vi "set_switch.vi"(8 "error in (no error)":errorcluster {"code" format="%.0x"}, 9 "switch":i32, 10 "topology name":T1="1127/2-Wire 32x1 Mux", 11 "resource name":refnum<k15>="SR" caption="switcher resource name") -> (0 "error out":errorcluster)   [LabVIEW 2016]
uses:
  <instrlib>/niSwitch/niSwitch.LLB/niSwitch Topologies.ctl
  <vilib>/DAQmx/configure/hardwareSpecific/Switch.llb/DAQmx Switch Connect (Single).vi
panel:
  out "Pixel Set?":bool
  out "instrument handle out":refnum<k15>="SC1Mod2 (7)"
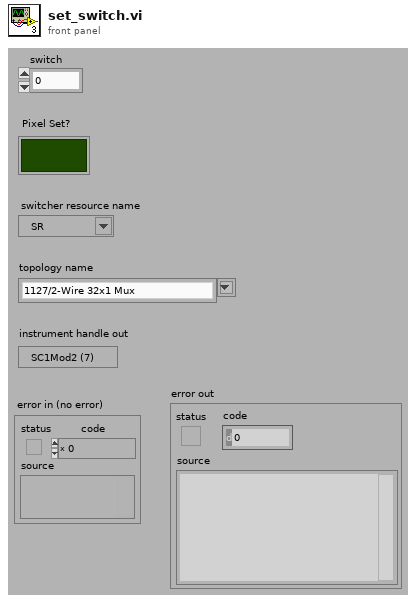
[diagram p1: front panel]
types:
  T1 = typedef "niSwitch Topologies.ctl" = string
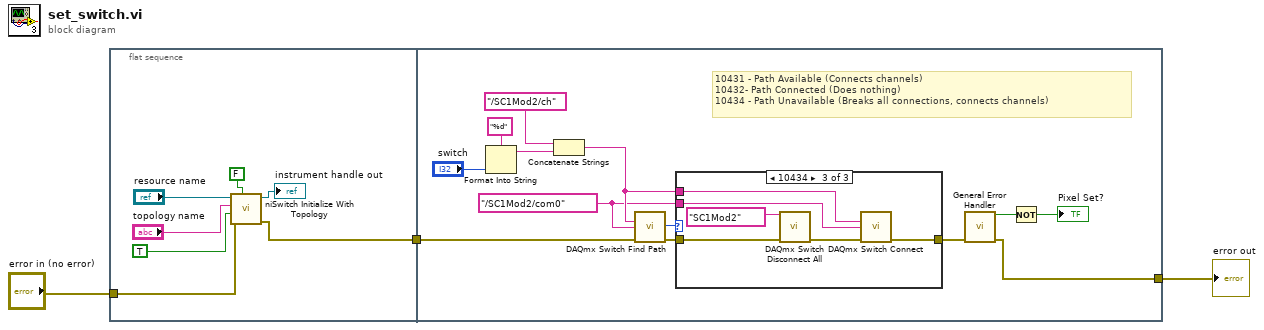
[diagram p0: block diagram]
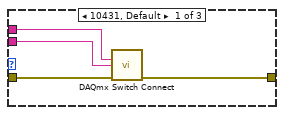
[diagram p2: hidden frame]
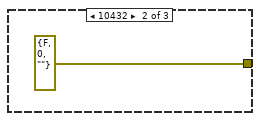
[diagram p3: hidden frame]
diagram:
  n1 = flat-sequence {
    tunnel: [w5] -> w3
    tunnel: "error in (no error)" -> [w4]
    tunnel: w3 -> [w12]
    tunnel: [w11] -> w1
    frame #0 {
      n2 = call <instrlib>:"niSwitch Initialize With Topology.vi"("simulate (boolean value)"=FALSE, "error in (no error)"=w4, "reset device (boolean value)"=TRUE, "topology name"="topology name", "resource name"="resource name") -> ("error out"=w5:errorcluster, "instrument handle out"=→"instrument handle out":refnum<k15>)  [unwired: 5 in]
    }
    frame #1 {
      w15 = tag "/SC1Mod2/com0" ("switch channel 1")
      # "10431 - Path Available (Connects channels)\n10432- Path Connected (Does nothing)\n10434 - Path Unavailable (Breaks all connections, connects channels)"
      n3 = Format Into String(format string="%d", "switch") -> (resulting string=w19:string)  [unwired: 2 in, 1 out]
      n4 = Concatenate Strings("/SC1Mod2/ch" ("resulting string"), w19) -> (w16:string)
      n5 = call <vilib>:"DAQmx Switch Find Path.vi"("switch channel 1"=w16, "switch channel 2"=w15, "error in"=w12) -> ("path status"=w17:i32, "error out"=w14:errorcluster)  [unwired: 10 in, 1 out]
      n6 = case shown="10434" w17 {
        tunnel: w16 -> [w27 _ w34]
        tunnel: w15 -> [w26 _ w29]
        tunnel: [w25 errorcluster {"status"=FALSE, "code"=0, "source"=""} ("error in (no error)") w32] -> w13
        tunnel: w14 -> [w24 _ w30]
        frame 10431, Default {
          n7 = call-poly <vilib>:"DAQmx Switch Connect.vi"("switch channel 1"=w27, "switch channel 2"=w26, "error in"=w24) -> ("error out"=w25:errorcluster)  [unwired: 12 in]
        }
        frame 10432 {
        }
        frame 10434 {
          n8 = call <vilib>:"DAQmx Switch Disconnect All.vi"("switch device"=tag "SC1Mod2", "error in"=w30) -> ("error out"=w33:errorcluster)  [unwired: 13 in]
          n9 = call-poly <vilib>:"DAQmx Switch Connect.vi"("switch channel 1"=w34, "switch channel 2"=w29, "error in"=w33) -> ("error out"=w32:errorcluster)  [unwired: 12 in]
        }
      }
      n10 = call <vilib>:"General Error Handler.vi"("error in (no error)"=w13) -> ("error?"=w23:bool, "error out"=w11:errorcluster)  [unwired: 10 in, 3 out]
      n11 = Not(x=w23) -> (.not. x?=→"Pixel Set?":bool)
    }
  }
  "error out" <- w1
